vi "Build Info.vi"(11 "Builder in":refnum<class "Builder.lvclass">) -> (2 "Build Info":T1[](array[typedef]), 3 "Builder out":refnum<class "Builder.lvclass">)   [LabVIEW 2020, in "Builder Tools.lvlib" / "Builder.lvclass"]
uses:
  Builder.lvclass
  Builder.lvclass/Builder.ctl
  Build Info.ctl
  Builder Tools.lvlib
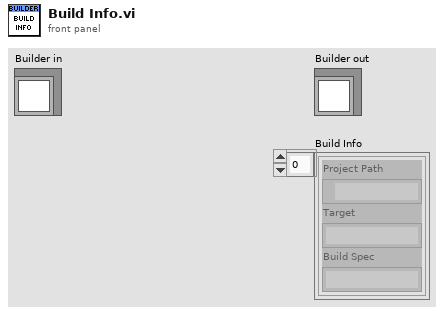
[diagram p1: front panel]
types:
  T1 = typedef "Builder Tools.lvlib/Build Info.ctl" = cluster{"Project Path":path, "Target":string, "Build Spec":string}
  T2 = typedef "Builder Tools.lvlib/Builder.lvclass/Build Step.ctl" = cluster{"Info":T1, "Build":refnum<class "Build.lvclass">}
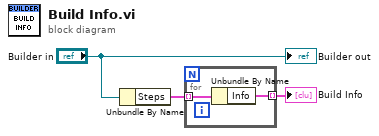
[diagram p0: block diagram]
diagram:
  n1 = Unbundle By Name("Builder in") -> ("Steps"=w2:T2[])
  n2 = for {
    tunnel: w2 -> [w5] mode=indexing
    tunnel: [w4] -> w1 mode=indexing
    n3 = Unbundle By Name(w5) -> ("Info"=w4:T1)
  }
  "Build Info" <- w1
  "Builder out" <- "Builder in"
